vi "LCA Read Pos Marker Counter.vi"(8 "error in (no error)":errorcluster caption="Fehler (Eingang, kein Fehler)", 11 "Axis Handle":i64) -> (0 "error out":errorcluster caption="Fehler (Ausgang)", 3 "Position Counter":u16)   [LabVIEW 2021, in "labbCAN_MotionControl_API.lvlib"]
doc: "LCA_Func long __stdcall LCA_ReadPosMarkerCounter(dev_hdl hAxis,\n unsigned short *pPosCounter);"
uses:
  labbCAN_MotionControl_API.lvlib
  labbCAN_MotionControl_API.dll
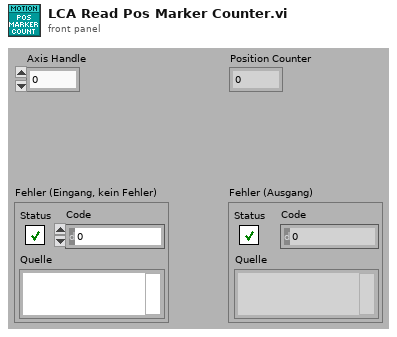
[diagram p1: front panel]
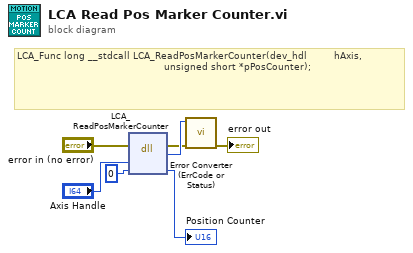
[diagram p0: block diagram]
diagram:
  # "LCA_Func long __stdcall LCA_ReadPosMarkerCounter(dev_hdl         hAxis,\n                                                 unsigned short *pPosCounter);"
  n1 = dll-call lib="C:/Users/olaja/AppData/Local/CETONI_SDK/labbCAN_MotionControl_API.*" fn="LCA_ReadPosMarkerCounter"(error in="error in (no error)", "hAxis"="Axis Handle", "pPosCounter"=u16 0) -> (error out=w2:errorcluster, "Rückgabetyp"=w7:i32, "pPosCounter"=→"Position Counter":u16)  [unwired: 3 in, 1 out]
  n2 = call "Error Converter (ErrCode or Status).vi"("error in (no error)"=w2, "error code"=w7) -> ("error out"=→"error out":errorcluster)  [unwired: 9 in]
